vi "Format VALUES (,,,).vi"(10 "Column Names":string[](array[string])=["Col1", "Col2", "Col3"], 11 "partial SQL":string="INSERT INTO ExampleTable") -> (3 "SQL":string caption="SQL+ (Col[]) VALUES (?[])")   [LabVIEW 2023, in "SQLiteSupport.lvlib"]
doc: "Formats an array, A, of column names into the form \"(A[0],A[1],...A[n]) VALUES (?,?...?)\". This is meant for creating an SQL INSERT statment from an array of column names that is ready to be bound to a matching array of values."
uses:
  SQLiteSupport.lvlib
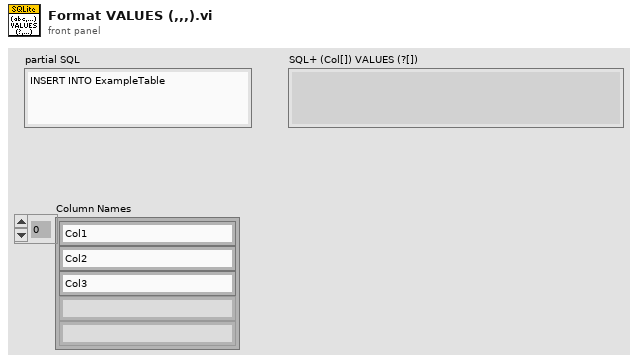
[diagram p1: front panel]
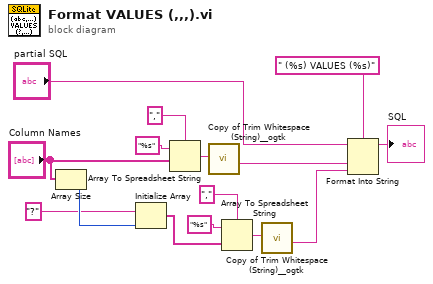
[diagram p0: block diagram]
diagram:
  n1 = Array Size(array="Column Names") -> (size(s)=w7:i32)
  n2 = Initialize Array("?", w7) -> (w3:string[])
  n3 = Array To Spreadsheet String(delimiter (Tab)=",", array="Column Names", 3:"%s" ("format string")) -> (spreadsheet string=w13:string)
  n4 = call "Copy of Trim Whitespace (String)__ogtk.vi"("String in"=w13) -> ("String out"=w12:string)  [unwired: 6 in]
  n5 = Array To Spreadsheet String(delimiter (Tab)=",", array=w3, 3:"%s" ("format string")) -> (spreadsheet string=w2:string)
  n6 = call "Copy of Trim Whitespace (String)__ogtk.vi"("String in"=w2) -> ("String out"=w1:string)  [unwired: 6 in]
  n7 = Format Into String(format string=" (%s) VALUES (%s)", initial string="partial SQL", w12, w1) -> (resulting string=→"SQL":string)  [unwired: 1 in, 1 out]
